vi "TalkTracker_low.vi"(0 "PORT NAME":string="Inlet_Heaters", 1 "Set":enum16{"Set", "Read"}(ring), 2 "Channel Name":string, 3 "Value to set":dbl, 5 "MODULE ADDRESS":i32=1, 9 "LOCATION":i32=15, 11 "NO. LOCATIONS":i32=1, 12 "Analogue":enum16{"Logic", "Analogue"}(ring), 13 "Timeout/ms":u32=500) -> (4 "Response":string=" ON\r\n", 10 "Set String":string, 15 "Comment out":string)   [LabVIEW 2010]
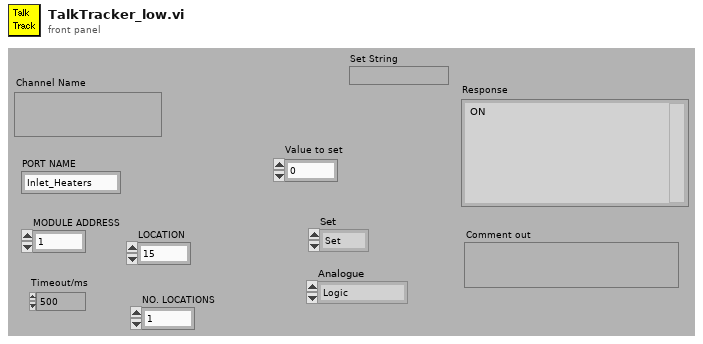
[diagram p1: front panel]
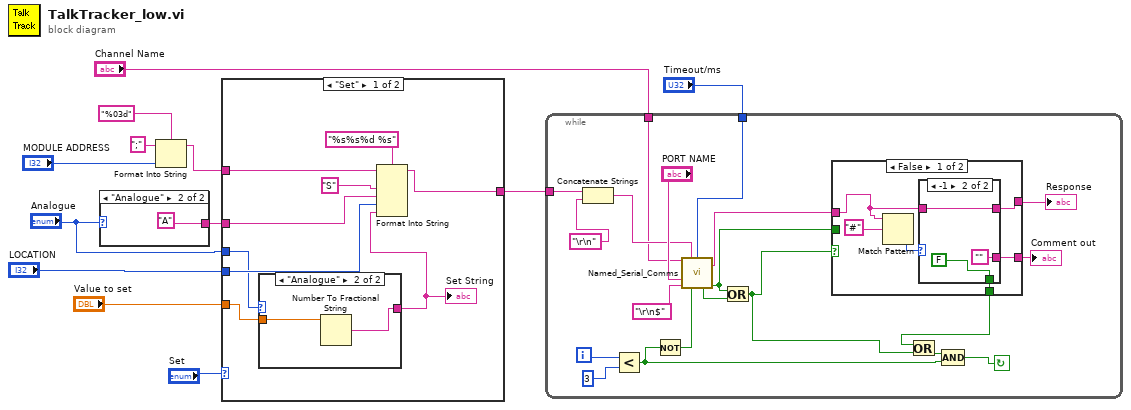
[diagram p0: block diagram]
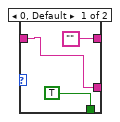
[diagram p2: hidden frame]
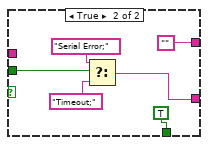
[diagram p3: hidden frame]
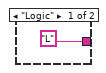
[diagram p4: hidden frame]
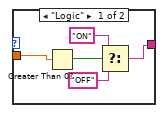
[diagram p5: hidden frame]
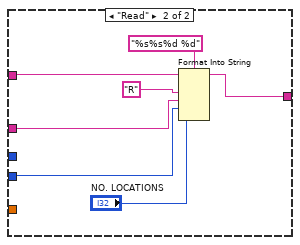
[diagram p6: hidden frame]
diagram:
  n1 = case shown="\"Analogue\"" "Analogue" {
    tunnel: ["L" "A" ("f")] -> w5
    frame "Logic" {
    }
    frame "Analogue" {
    }
  }
  n2 = Format Into String(format string="%03d", initial string=";", "MODULE ADDRESS") -> (resulting string=w9:string)  [unwired: 1 in, 1 out]
  n3 = case shown="\"Set\"" "Set" {
    tunnel: w9 -> [w23 w37]
    tunnel: "LOCATION" -> [w22 w34]
    tunnel: [w21 w32] -> w7
    tunnel: "Value to set" -> [w16 _]
    tunnel: w5 -> [w18 w31]
    tunnel: "Analogue" -> [w17 _]
    frame "Set" {
      n4 = case shown="\"Analogue\"" w17 {
        tunnel: [w26 w29] -> w15
        tunnel: w16 -> [w28 w30]
        frame "Logic" {
          n5 = Greater Than 0?(x=w28) -> (x > 0?=w27:bool)
          n6 = Select(t="ON", s=w27, f="OFF") -> (s? t:f=w26:string)
        }
        frame "Analogue" {
          n7 = Number To Fractional String(number=w30) -> (F-format string=w29:string)  [unwired: 3 out]
        }
      }
      "Set String" <- w15
      n8 = Format Into String(format string="%s%s%d %s", initial string=w23, "S", w18, w22, w15) -> (resulting string=w21:string)  [unwired: 1 in, 1 out]
    }
    frame "Read" {
      n9 = Format Into String(format string="%s%s%d %d", initial string=w37, "R", w31, w34, "NO. LOCATIONS") -> (resulting string=w32:string)  [unwired: 1 in, 1 out]
    }
  }
  n10 = while {
    tunnel: w7 -> [w54]
    tunnel: "Channel Name" -> [w52]
    tunnel: "Timeout/ms" -> [w38]
    i -> [w47]
    stop <- w49 continue-if-true
    n11 = Concatenate Strings(w54, "\r\n" ("Term Grep")) -> (w53:string)
    n12 = Less?(x=w47, y=3) -> (x < y?=w40:bool)
    n13 = Not(x=w40) -> (.not. x?=w39:bool)
    n14 = call "Named_Serial_Comms.vi"("Channel Name"=w52, "Write String"=w53, "Timeout/ms"=w38, "Port Name"="PORT NAME", "Term Grep"="\r\n$", "Log Errors?"=w39) -> ("Read"=w44:string, "Timed out"=w51:bool, "Serial Error"=w50:bool)  [unwired: 3 in, 4 out]
    n15 = Or(x=w50, y=w51) -> (x .or. y?=w42:bool)
    n16 = case shown="False" w42 {
      tunnel: w44 -> [w60 _]
      tunnel: [w61 w74] -> w45
      tunnel: [w59 ""] -> w46
      tunnel: w50 -> [_ w75]
      tunnel: [w58 TRUE] -> w43
      frame False {
        n17 = Match Pattern(string=w60, regular expression="#") -> (offset past match=w62:i32)  [unwired: 4 out]
        n18 = case shown="-1" w62 {
          tunnel: [w64 ""] -> w61
          tunnel: w60 -> [w64 w68]
          tunnel: ["" w68] -> w59
          tunnel: [TRUE FALSE] -> w58
          frame 0, Default {
          }
          frame -1 {
          }
        }
      }
      frame True {
        n19 = Select(t="Serial Error;", s=w75, f="Timeout;") -> (s? t:f=w74:string)
      }
    }
    "Response" <- w46
    "Comment out" <- w45
    n20 = Or(x=w43, y=w42) -> (x .or. y?=w41:bool)
    n21 = Compound Arithmetic op=AND(w41, w40) -> (w49:bool)
  }
